vi "ExInitTestGlobal.vi"() -> ()   [LabVIEW 2010]
uses:
  GlbCamHndls.vi
panel:
  in  "Number of Spectrometers":u32=1 min=1 step=1
  out "error out":errorcluster
  in  "error in (no error)":errorcluster
  in  "Number of Cameras":u32=1 min=1 step=1
  # "ExInitTestGlobal.vi : initialize and open n number of \ncameras and spectrometers. The handles are stored\nin global variables for later use."
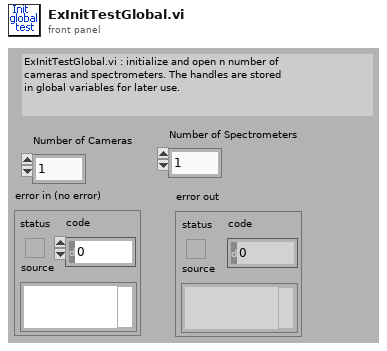
[diagram p1: front panel]
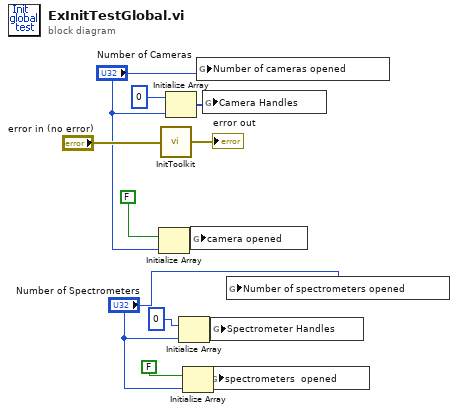
[diagram p0: block diagram]
diagram:
  n1 = Initialize Array(FALSE, "Number of Cameras") -> (w6:bool[])
  n2 = call <userlib>:"InitToolkit.vi"("error in"="error in (no error)") -> ("error out"=→"error out":errorcluster)
  n3 = Initialize Array(0, "Number of Cameras") -> (w10:i32[])
  n4 = Initialize Array(0, "Number of Spectrometers") -> (w2:i32[])
  n5 = Initialize Array(FALSE, "Number of Spectrometers") -> (w1:bool[])
  n6 = global write "GlbCamHndls.vi" "camera opened"(w6) -> ()
  n7 = global write "GlbCamHndls.vi" "Number of cameras opened"("Number of Cameras") -> ()
  n8 = global write "GlbCamHndls.vi" "Camera Handles"(w10) -> ()
  n9 = global write "GlbCamHndls.vi" "spectrometers  opened"(w1) -> ()
  n10 = global write "GlbCamHndls.vi" "Spectrometer Handles"(w2) -> ()
  n11 = global write "GlbCamHndls.vi" "Number of spectrometers opened"("Number of Spectrometers") -> ()
